vi "NI6602.destructor.vi"(0 "i ref in":refnum<vi>, 5 "error in (no error)":errorcluster) -> (19 "error out":errorcluster)   [LabVIEW 2014, in "NI6602.lvlib"]
doc: "This is the destructor of a class.\n\nLicense Agreement for this software:\n\nCopyright (C)\nGesellschaft für Schwerionenforschung, GSI\nPlanckstr. 1\n64291 Darmstadt\nGermany\n\nContact: D.Beck@gsi.de \n\nThis program is free software; you can redistribute it and/or modify it under the terms of the \nGNU General Public License as published by the Free Software Foundation; either version 2 of \nthe license, or (at your option) any later version.\n\nThis program is distributed in the hope that it will be useful, but WITHOUT ANY WARRANTY; \nwithout even the implied warranty of MERCHANTABILITY or FITNESS FOR A PARTICULAR PURPOSE. See the GNU General License for more details (http://www.gnu.org).\n\nGesellschaft für Schwerionenforschung, GSI\nPlanckstr. 1, 64291 Darmstadt, Germany\nFor all questions and ideas contact: M.Richter@gsi.de, H.Brand@gsi.de or D.Beck@gsi.de.\nLast update: 16-JUN-2004"
uses:
  NI6602.lvlib
  CS_Core/CSApplicationBaseClasses/DeviceBase/DeviceBase.lvlib
  CSlibraries-extern/DimLVEvent/LVDimInterface/LVDimInterface.lvlib
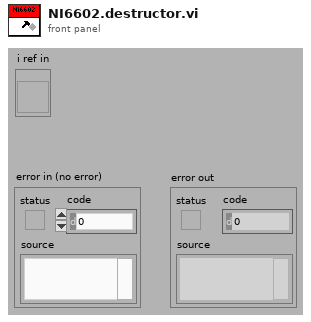
[diagram p1: front panel]
types:
  T1 = typedef "NI6602.lvlib/NI6602.i attribute.ctl" = cluster{"CounterDAQ Channels":cluster{"task":refnum<k21>, "Channel Name":string}[], "RateServiceIDs":i32[], "Running?":bool, "IntegralServiceIDs":i32[], "ThresholdID":i32, "Threshold":dbl, "IntegralValues":dbl[], "Stopped?":bool}
  T2 = enum16{"SetAttribute", "GetAttribute", "CreateAttribute", "DestroyAttribute", "DestroyAllAtributes"}
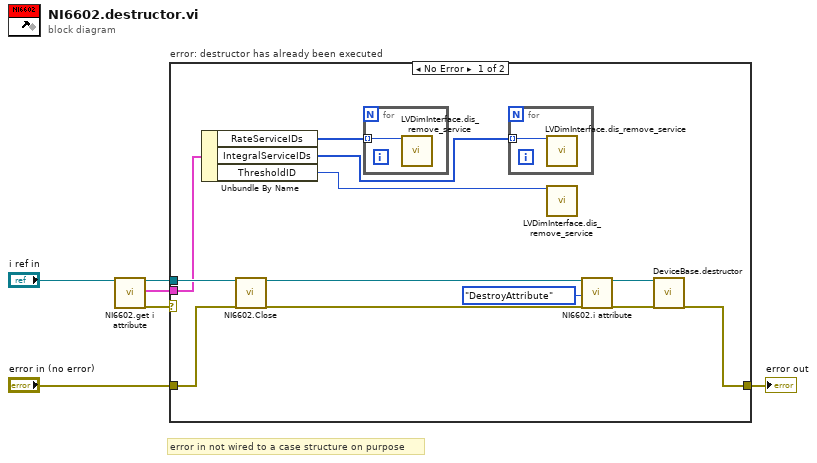
[diagram p0: block diagram]
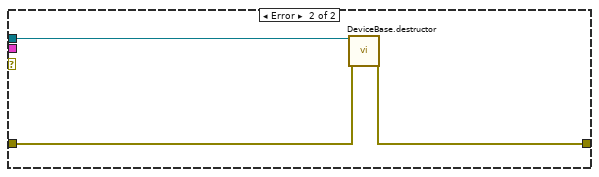
[diagram p2: hidden frame]
diagram:
  # "error in not wired to a case structure on purpose"
  n1 = call "NI6602.get i attribute.vi"("i ref in"="i ref in") -> ("i ref out"=w2:refnum<vi>, "i attribute"=w1:T1, "error out"=w3:errorcluster)  [unwired: 16 in]
  n2 = case "error: destructor has already been executed" shown="No Error" w3 {
    tunnel: [w15 w21] -> w6
    tunnel: "error in (no error)" -> [w14 w22]
    tunnel: w2 -> [w11 w23]
    tunnel: w1 -> [w10 _]
    frame No Error {
      n3 = Unbundle By Name(w10) -> ("RateServiceIDs"=w9:i32[], "IntegralServiceIDs"=w8:i32[], "ThresholdID"=w7:i32)
      n4 = call "NI6602.Close.vi"("i ref in"=w11, "error in (no error)"=w14) -> ("i ref out"=w12:refnum<vi>, "error out"=w13:errorcluster)  [unwired: 16 in]
      n5 = for {
        tunnel: w9 -> [w20] mode=indexing
        n6 = call "LVDimInterface.dis_remove_service.vi"("my_serviceID"=w20) -> ()  [unwired: 18 in, 1 out]
      }
      n7 = for {
        tunnel: w8 -> [w19] mode=indexing
        n8 = call "LVDimInterface.dis_remove_service.vi"("my_serviceID"=w19) -> ()  [unwired: 18 in, 1 out]
      }
      n9 = call "LVDimInterface.dis_remove_service.vi"("my_serviceID"=w7) -> ()  [unwired: 18 in, 1 out]
      n10 = call "NI6602.i attribute.vi"("VI Refnum"=w12, "Action"=T2."DestroyAttribute", "error in (no error)"=w13) -> ("VI Refnum out"=w17:refnum<vi>, "error out"=w16:errorcluster)  [unwired: 14 in, 1 out]
      n11 = call "DeviceBase.destructor.vi"("i ref in"=w17, "error in (no error)"=w16) -> ("error out"=w15:errorcluster)  [unwired: 17 in]
    }
    frame Error {
      n12 = call "DeviceBase.destructor.vi"("i ref in"=w23, "error in (no error)"=w22) -> ("error out"=w21:errorcluster)  [unwired: 17 in]
    }
  }
  "error out" <- w6
